vi "overlay_axis(subVI).vi"(8 "error in (no error)":errorcluster, 10 "image dst":T1, 11 "image src":T1) -> (0 "error out":errorcluster, 2 "Origin Pixel":cluster{"X":sgl, "Y":sgl}, 3 "Image Out":T1)   [LabVIEW 2020]
doc: "Disegna il sistema di riferimento da un'immagine già calibrata. Richiede in ingresso un'immagine calibrata (image src) mentre image dst è dove si vuole fare l'overlay. Fornisce in uscita anche le cordinate del sistema di riferimento."
uses:
  <vilib>/vision/Image Controls.llb/IMAQ Image.ctl
  <vilib>/vision/NI_Vision_Development_Module.lvlib
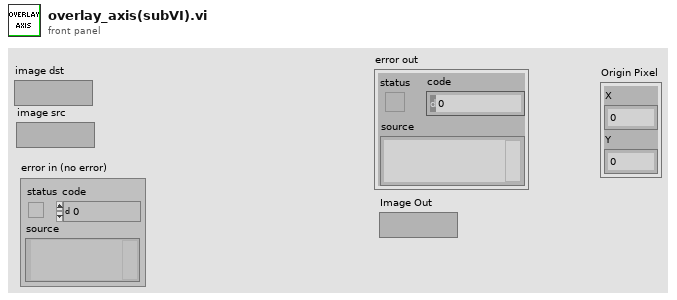
[diagram p1: front panel]
types:
  T1 = typedef "IMAQ Image.ctl" = refnum<image>
  T2 = cluster{"Origin Pixel":cluster{"X":sgl, "Y":sgl}, "Angle Relative to Horizontal (deg)":sgl, "Axis Reference":u32}
  T3 = cluster{"Origin Pixel":cluster{"X":sgl, "Y":sgl}, "Angle Relative to Horizontal (deg)":sgl, "X Axis Pixel":cluster{"X":sgl, "Y":sgl}, "Axis Reference":u32}
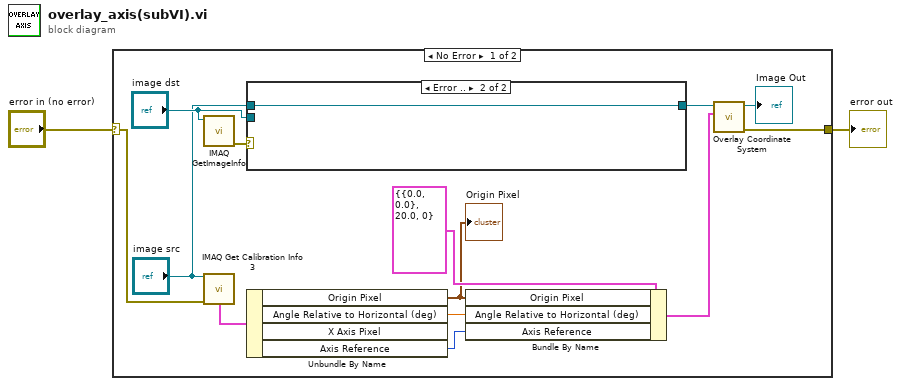
[diagram p0: block diagram]
diagram:
  n1 = case shown="No Error" "error in (no error)" {
    selector: "error in (no error)" -> [w12 w18]
    tunnel: [w3 w18] -> w2
    frame No Error {
      n2 = call "IMAQ GetImageInfo"("Image"="image dst") -> ("error out"=w7:errorcluster)  [unwired: 3 in, 7 out]
      n3 = call "IMAQ Get Calibration Info 3"("Calibration Template Image"="image src", "error in (no error)"=w12) -> ("Calibration Axis Info"=w11:T3)  [unwired: 5 in, 8 out]
      n4 = case shown="Error .." w7 {
        tunnel: [w16 w17] -> w6
        tunnel: "image dst" -> [w16 _]
        tunnel: "image src" -> [_ w17]
        frame No Error {
        }
        frame Error {
        }
      }
      n5 = Unbundle By Name(w11) -> ("Origin Pixel"=w9:cluster{"X":sgl, "Y":sgl}, "Angle Relative to Horizontal (deg)"=w8:sgl, "Axis Reference"=w10:u32)  [unwired: 1 out]
      "Origin Pixel" <- w9
      n6 = Bundle By Name(cluster=T2 {"Origin Pixel"={"X"=0.0, "Y"=0.0}, "Angle Relative to Horizontal (deg)"=20.0, "Axis Reference"=0} ("Calibration Axis Info"), "Origin Pixel"=w9, "Angle Relative to Horizontal (deg)"=w8, "Axis Reference"=w10) -> (w14:T2)
      n7 = call "Overlay Coordinate System.vi"("Calibration Axis Info"=w14, "Image"=w6) -> ("error out"=w3:errorcluster, "Image Out"=→"Image Out":T1)  [unwired: 8 in]
    }
    frame Error {
    }
  }
  "error out" <- w2
